vi "VALEW_ATC_Calc Segment Target Temp.vi"(0 "T(target)":dbl, 5 "V(bath)":dbl, 9 "V(segment)":dbl, 11 "T(bath)":dbl) -> (8 "T(segment target)":dbl)   [LabVIEW 2016, in "2015 VA Washer.lvlib"]
uses:
  Projects/2015 VA Washer.lvlib
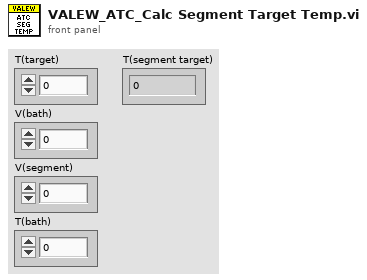
[diagram p1: front panel]
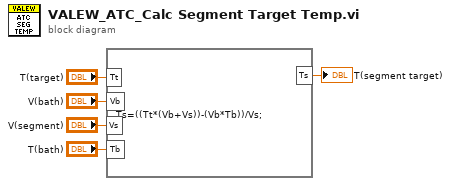
[diagram p0: block diagram]
diagram:
  n1 = formula code="Ts=((Tt*(Vb+Vs))-(Vb*Tb))/Vs;"("Tt"="T(target)", "Vb"="V(bath)", "Vs"="V(segment)", "Tb"="T(bath)") -> ("Ts"=→"T(segment target)":dbl)
